vi "add PID Element to PID Array.vi"(8 "error in":errorcluster, 10 "PID Element":T1={"Loop ID"="", "Tags"={"Setpoint"="", "Process Variable"="", "Output"=""}, "Gains"={"P"=1.0, "I"=0.01, "D"=0.0}, "Range"={"High"=100.0, "Low"=-100.0}}, 11 "PID Array ref in":T2) -> (0 "error out":errorcluster)   [LabVIEW 2015, in "PID Module editor node.lvclass"]
doc: "This VI takes in a reference to a PID Array and adds a PID Element to it"
uses:
  PID Module editor node.lvclass
  PID array reference.ctl
  PID array element.ctl
  module/configuration/PID Module configuration.lvclass
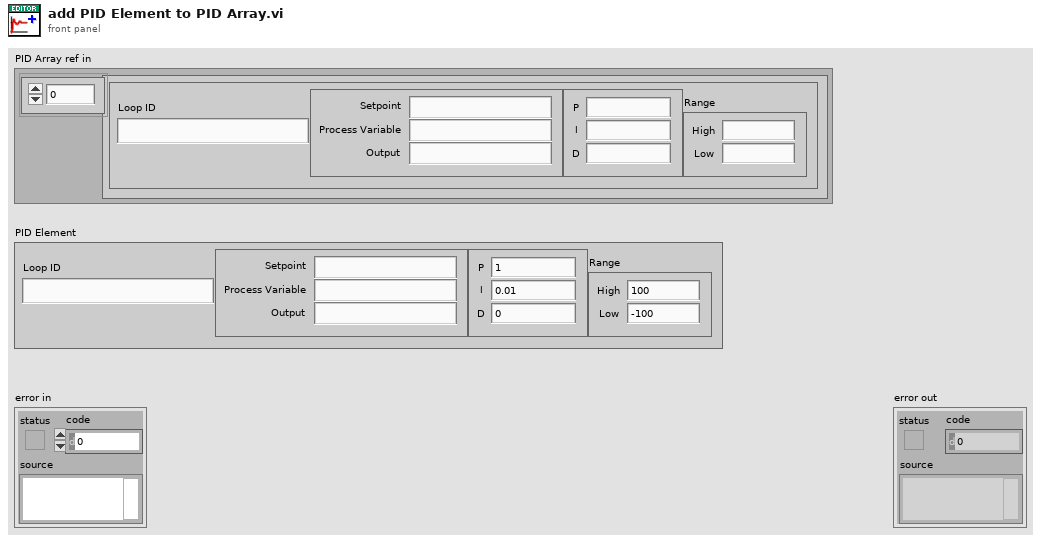
[diagram p1: front panel]
types:
  T1 = typedef "PID Module configuration.lvclass/PID array element.ctl" = cluster{"Loop ID":string, "Tags":cluster{"Setpoint":string, "Process Variable":string, "Output":string}, "Gains":cluster{"P":dbl, "I":dbl, "D":dbl}, "Range":cluster{"High":dbl, "Low":dbl}}
  T2 = typedef "PID Module editor node.lvclass/PID array reference.ctl" = refnum<vi>
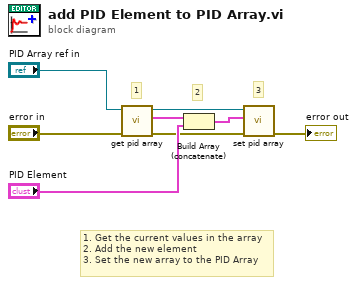
[diagram p0: block diagram]
diagram:
  # "1. Get the current values in the array\n2. Add the new element\n3. Set the new array to the PID Array"
  # "3"
  # "2"
  # "1"
  n1 = call "get pid array.vi"("error in (no error)"="error in", "Array in"="PID Array ref in") -> ("error out"=w2:errorcluster, "Value"=w7:T1[], "Array out"=w1:T2)  [unwired: 7 in]
  n2 = Build Array (concatenate)(w7, "PID Element") -> (w5:T1[])
  n3 = call "set pid array.vi"("error in (no error)"=w2, "Array"=w5, "Array in"=w1) -> ("error out"=→"error out":errorcluster)  [unwired: 7 in, 1 out]
